vi "Reading Frequency.vi"(8 "error in":errorcluster, 11 "Tlcu Temp":dbl format="%#_12f") -> (0 "Error Out":errorcluster, 1 "Pass/Fail":bool, 2 "Adj Factor":u8[](array[numeric]) format="%x", 3 "MeasuredFreq_1":dbl format="%#_12f")   [LabVIEW 2009]
uses:
  <vilib>/Instr/_visa.llb/VISA Configure Serial Port (Instr).vi
  Global/Global 1.vi
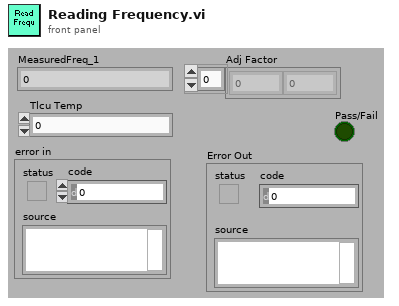
[diagram p1: front panel]
types:
  T1 = enum16{"Write then Read", "Write to Instr", "Read from Instr"}
  T2 = cluster{"VHEATFUSENOLOADMIN":string, "VHEATFUSELOADMAX":string, "VOVERRIDEDIODEMIN":string, "TDIFFMAX":string, "MEASFREQMAX":string, "MEASFREQMIN":string, "VOVER":string, "VMIDDLE":string, "VUNDER":string, "VNORESET":string, "VRESET":string, "WAITPING":string, "LRFID":string, "RFIDUID":string, "EXTEESIZE":string, "LCUTYPE":string, "LCUSUBTYPE":string, "TEVN":string, "BOOTVER":string, "APPVER":string, "ISLEEPMAX":string, "TSLEEP":string, "APPWAIT":string, "DBWAIT":string}
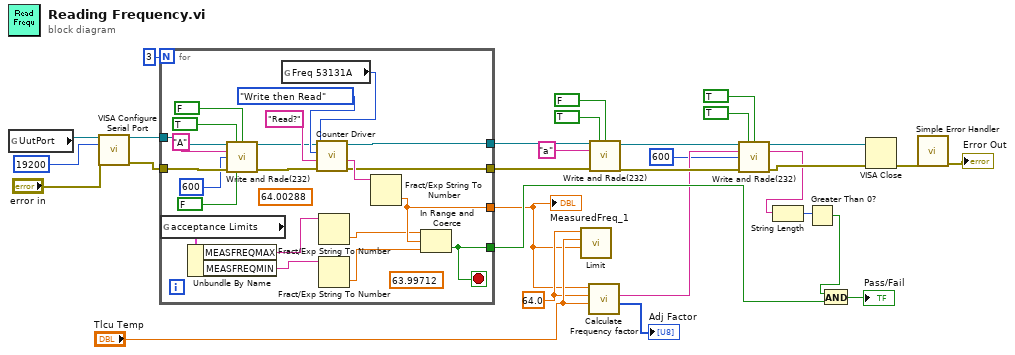
[diagram p0: block diagram]
diagram:
  w16 = 64.0 ("OkFreq")
  n1 = global read "Global 1.vi" "UutPort"() -> (w29:refnum<visa-resource-name>)
  n2 = call-poly "VISA Configure Serial Port"("VISA resource name"=w29, "baud rate (9600)"=u32 19200 ("baud rate(read)"), "error in (no error)"="error in") -> ("VISA resource name out"=w26:refnum<visa-resource-name>, "error out"=w25:errorcluster)  [unwired: 3 in, 8 out]
  n3 = for {
    N: 3 -> [_]
    tunnel: [w39] -> w9
    tunnel: [w47] -> w12
    tunnel: w26 -> [w43]
    tunnel: w25 -> [w42]
    tunnel: [w41] -> w11
    tunnel: [w38] -> w17
    stop <- w38 stop-if-true
    (unwired) 63.99712 ("lower limit")
    (unwired) 64.00288 ("upper limit")
    n4 = global read "Global 1.vi" "acceptance Limits"() -> (w35:T2)
    n5 = Unbundle By Name(w35) -> ("MEASFREQMAX"=w34:string, "MEASFREQMIN"=w33:string)
    n6 = call "Write and Rade(232).vi"("VISA resource name in"=w43, "write"=TRUE, "read"=FALSE, "string to write"="A", "ms delay"=u32 600 ("millisecond multiple"), "error in"=w42, "change baud rate(read)"=FALSE) -> ("VISA resource name out"=w41:refnum<visa-resource-name>, "error out"=w40:errorcluster)  [unwired: 1 in, 6 out]
    n7 = global read "Global 1.vi" "Freq 53131A"() -> (w51:u32)
    n8 = call "Counter Driver.vi"("error in"=w40, "Characters to Write"="Read?", "Operation"=T1."Write then Read", "GPIB Address"=w51) -> ("Error Out"=w47:errorcluster, "Characters Read"=w48:string)  [unwired: 6 out]
    n9 = Fract/Exp String To Number(string=w34) -> (number=w31:dbl)  [unwired: 4 out]
    n10 = Fract/Exp String To Number(string=w33) -> (number=w32:dbl)  [unwired: 4 out]
    n11 = Fract/Exp String To Number(string=w48) -> (number=w39:dbl)  [unwired: 4 out]
    n12 = In Range and Coerce(upper limit=w31, x=w39, lower limit=w32) -> (In Range?=w38:bool)  [unwired: 1 out]
  }
  "MeasuredFreq_1" <- w9
  n13 = call "Limit.vi"("MeasuredFreq"=w9, "TLcu"="Tlcu Temp", "OkFreq"=w16) -> ()  [unwired: 9 out]
  n14 = call "Calculate Frequency factor.vi"("TLcu"="Tlcu Temp", "OkFreq"=w16, "MeasuredFreq"=w9) -> (1:"Adj Factor"=→"Adj Factor":u8[], 2:"Adj Factor"=w8:string)  [unwired: 7 out]
  n15 = call "Write and Rade(232).vi"("VISA resource name in"=w11, "write"=TRUE, "read"=FALSE, "string to write"="a", "error in"=w12) -> ("VISA resource name out"=w20:refnum<visa-resource-name>, "error out"=w19:errorcluster)  [unwired: 3 in, 6 out]
  n16 = call "Write and Rade(232).vi"("VISA resource name in"=w20, "write"=TRUE, "read"=TRUE, "string to write"=w8, "ms delay"=u32 600 ("millisecond multiple"), "error in"=w19) -> ("VISA resource name out"=w6:refnum<visa-resource-name>, "read string"=w3:string, "error out"=w5:errorcluster)  [unwired: 2 in, 5 out]
  n17 = String Length(string=w3) -> (length=w2:i32)
  n18 = Greater Than 0?(x=w2) -> (x > 0?=w1:bool)
  n19 = And(x=w1, y=w17) -> (x .and. y?=→"Pass/Fail":bool)
  n20 = VISA Close(VISA resource name=w6, error in (no error)=w5) -> (error out=w24:errorcluster)
  n21 = call <vilib>:"Simple Error Handler.vi"("error in (no error)"=w24) -> ("error out"=→"Error Out":errorcluster)  [unwired: 1 in, 7 out]
